vi "VisualMonitoring.vi"(8 "error in":errorcluster) -> ()   [LabVIEW 2014]
uses:
  Gantry/GantryGlobals.vi
  <vilib>/Rock Robotics/Network Tables/SD Write Numeric Array.vi
panel:
  out "Lift Setpoint":dbl
  out "Tote Sense 2":bool
  out "LiftSetpoint":dbl
  out "Gyro Angle":dbl
  out "Tote Sense":bool
  out "Front Left Wheel Encoder Position":dbl
  out "Front Left Wheel":dbl(graph)
  out "Right Arm Lift Velocity":dbl(graph)
  out "Left Arm Lift Velocity":dbl(graph)
  out "LiftError":dbl
  out "Closed Loop Error Gantry":dbl
  out "Closed Loop Error LiftL":dbl
  out "Closed Loop Error ArmR":dbl
  out "Closed Loop Error LiftR":dbl
  out "Closed Loop Error ArmL":dbl
  out "Left Arm Applied Throttle":dbl
  out "Right Arm Applied Throttle":dbl
  out "Encoder Position FL":dbl=414.0
  out "Applied Throttle FL":dbl
  out "Encoder Position FR":dbl=414.0
  out "Applied Throttle FR":dbl
  out "Encoder Position BL":dbl=414.0
  out "Applied Throttle BL":dbl
  out "Encoder Position BR":dbl=414.0
  out "Applied Throttle BR":dbl
  out "Closed Loop Error FL":dbl
  out "Closed Loop Error FR":dbl
  out "Closed Loop Error BL":dbl
  out "Closed Loop Error BR":dbl
  out "Right Lift":cluster{"FL Angle":dbl, "Encoder Position":dbl}(graph)={"FL Angle"=0.0, "Encoder Position"=1.0}
  out "Left Lift":cluster{"FL Angle":dbl, "Encoder Position":dbl}(graph)={"FL Angle"=2.0, "Encoder Position"=1.0}
  out "Gantry":cluster{"FL Angle":dbl, "Encoder Position":dbl}(graph)={"FL Angle"=2019.0, "Encoder Position"=2100.0}
  out "Left Arm":cluster{"FL Angle":dbl, "Encoder Position":dbl}(graph)
  out "Right Arm":cluster{"FL Angle":dbl, "Encoder Position":dbl}(graph)
  out "Gantry Position":dbl=2019.0
  out "Gantry Applied Throttle":dbl
  out "Lift Encoder R":dbl
  out "Lift Encoder L":dbl
  out "Right Lift Throttle":dbl
  out "Left Lift Throttle":dbl
  out "Left Arm Position":dbl
  out "Right Arm Position":dbl
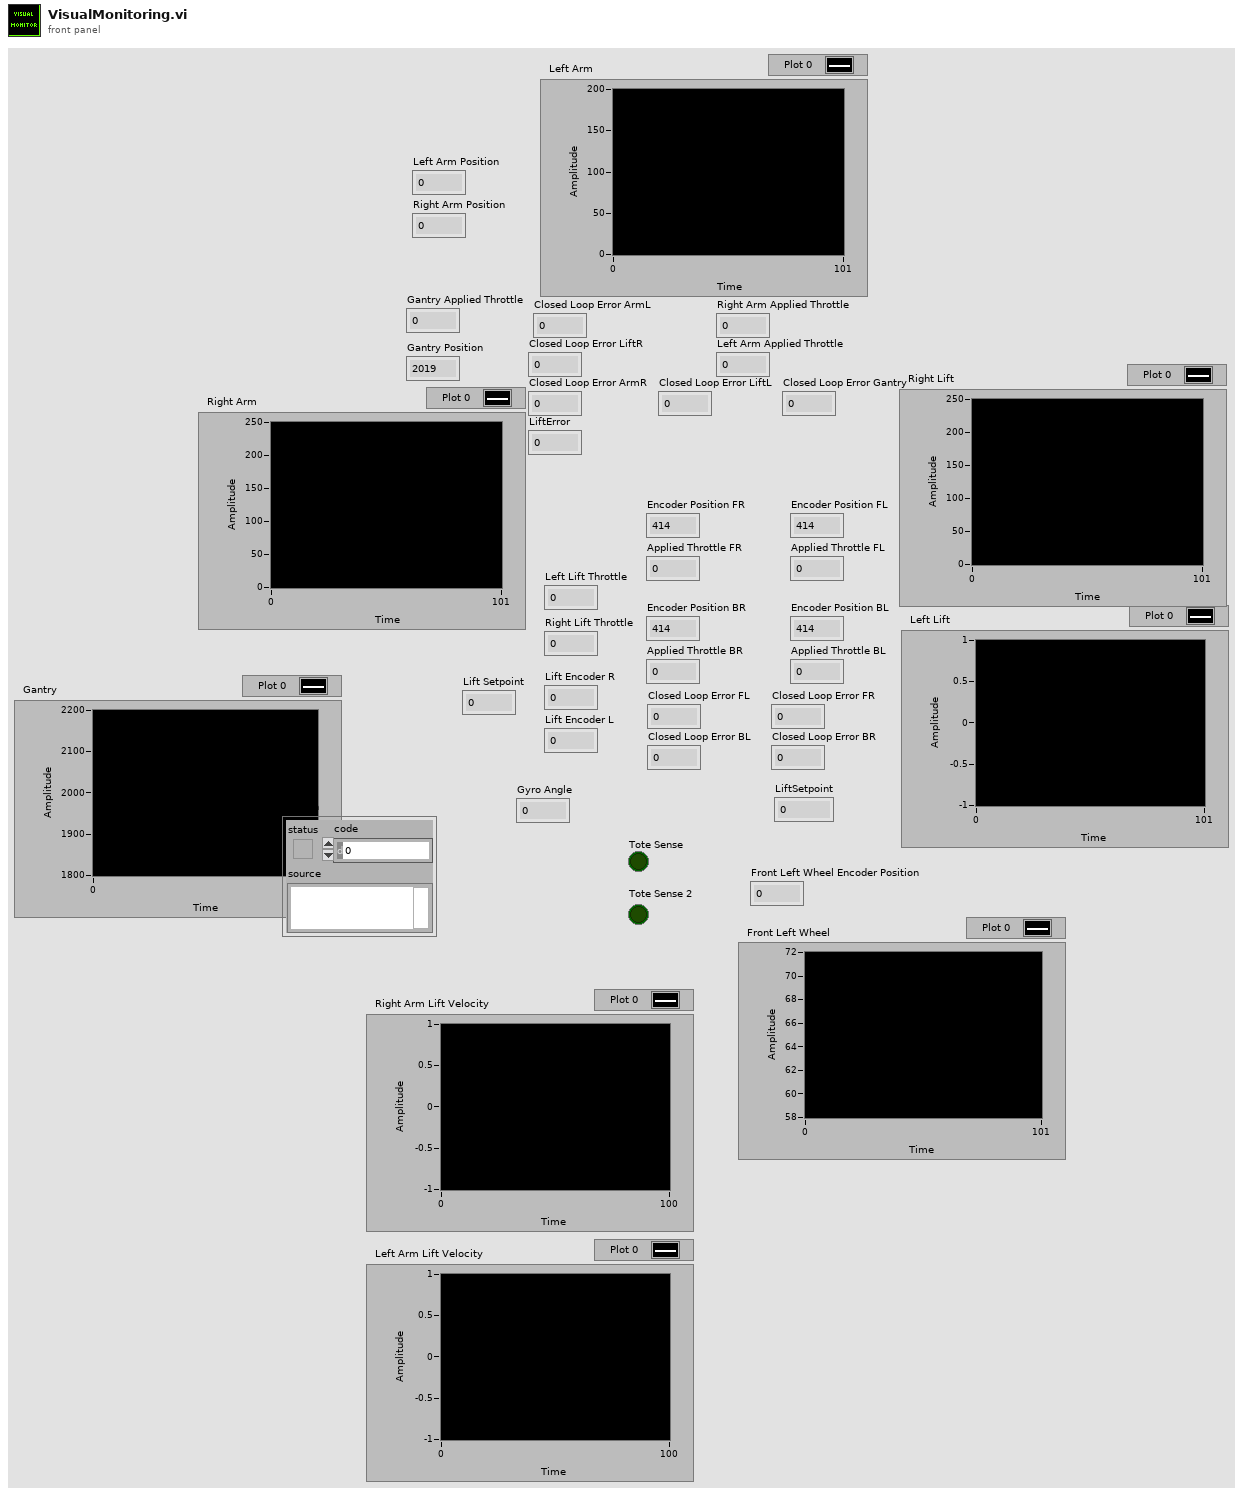
[diagram p1: front panel]
types:
  T1 = typedef "WPI_AccelerometerDevRef.ctl" = cluster{"DevStatus":errorcluster, "Controller":T2, "Scaling":T3, "Analog Channels":T4, "I2C Bus":T6, "SPI Bus":T7, "Accel Range":T8, "ADXL345 Axes":T9, "Handle":i32, "Device Address":u8, "Accel Type":enum16{"Analog", "ADXL345 I2C", "ADXL345 SPI", "Internal"}}
  T2 = typedef "FPGA_TypedefAnalogModule.ctl" = enum16{"Controller 1"}
  T3 = typedef "WPI_AccelerometerScaling.ctl" = cluster{"Gain (VoltsPerG)":dbl, "Center Voltage":dbl}
  T4 = typedef "WPI_AccelerometerAnalogChannels.ctl" = cluster{"X-Axis":T5, "Y-Axis":T5, "Z-Axis":T5}
  T5 = typedef "FPGA_AIChannel.ctl" = enum8{"AI 0", "AI 1", "AI 2", "AI 3", "AI MXP 0", "AI MXP 1", "AI MXP 2", "AI MXP 3", "Invalid"}
  T6 = typedef "i2c_bus.ctl" = enum16{"I2C On-Board", "I2C MXP", "Invalid"}
  T7 = typedef "spi_bus.ctl" = enum16{"SPI On-Board, CS0", "SPI On-Board, CS1", "SPI On-Board, CS2", "SPI On-Board, CS3", "SPI MXP", "Invalid"}
  T8 = typedef "ADXL345 Range.ctl" = u8
  T9 = typedef "WPI_AccelerometerADXL345 Axes.ctl" = cluster{"X-Axis":bool, "Y-Axis":bool, "Z-Axis":bool}
  T10 = cluster{"X-Axis":dbl, "Y-Axis":dbl, "Z-Axis":dbl}
  T11 = typedef "WPI_JoystickDevRef.ctl" = cluster{"Device":T12}
  T12 = typedef "WPI_JoystickDeviceEnum.ctl" = enum16{"USB 0", "USB 1", "USB 2", "USB 3", "USB 4", "USB 5"}
  T13 = typedef "WPI_SwitchDevRef.ctl" = cluster{"DevStatus":errorcluster, "DIO Channel":T14, "Controller":T15, "CntIndex":T16, "Normally Closed":bool}
  T14 = typedef "FPGA_DIOChannel.ctl" = enum8{"DIO 0", "DIO 1", "DIO 2", "DIO 3", "DIO 4", "DIO 5", "DIO 6", "DIO 7", "DIO 8", "DIO 9", "DIO MXP 0", "DIO MXP 1", "DIO MXP 2", "DIO MXP 3", "DIO MXP 4", "DIO MXP 5", "DIO MXP 6", "DIO MXP 7", "DIO MXP 8", "DIO MXP 9", "DIO MXP 10", "DIO MXP 11", "DIO MXP 12", "DIO MXP 13", "DIO MXP 14", "DIO MXP 15", "Invalid"}
  T15 = typedef "FPGA_TypedefDigitalModule.ctl" = enum16{"Controller 1"}
  T16 = typedef "FPGA_CounterCtrSystemIndex.ctl" = enum8{"Ctr 0", "Ctr 1", "Ctr 2", "Ctr 3", "Ctr 4", "Ctr 5", "Ctr 6", "Ctr 7", "Invalid"}
  T17 = typedef "WPI_GyroDevRef.ctl" = cluster{"DevStatus":errorcluster, "Analog Module":T2, "Analog Channel":T5, "Offset":dbl, "Gain (VoltsPerDegree/Second)":dbl}
  T18 = typedef "WPI_MotorControlDeviceRef.ctl" = cluster{"DeviceStatus":errorcluster, "Type":T19, "PWM":cluster{"Controller":T15, "PWM Channel":T20, "DeadBand":T21}, "CAN":cluster{"Device Number":u8, "Control Mode":T22, "Semaphore":T23, "Max Vout":dbl, "TalonSRX Control Mode":T24}, "Invert":bool, "TransformRef":T25, "InvTransformRef":T25}
  T19 = typedef "WPI_MotorControlType.ctl" = enum16{"PWM", "CAN", "CANTalonSRX"}
  T20 = typedef "FPGA_DIOPWMChannel.ctl" = enum8{"PWM 0", "PWM 1", "PWM 2", "PWM 3", "PWM 4", "PWM 5", "PWM 6", "PWM 7", "PWM 8", "PWM 9", "PWM MXP 0", "PWM MXP 1", "PWM MXP 2", "PWM MXP 3", "PWM MXP 4", "PWM MXP 5", "PWM MXP 6", "PWM MXP 7", "PWM MXP 8", "PWM MXP 9", "Invalid"}
  T21 = typedef "WPI_PWMDeadband.ctl" = cluster{"Name":string, "maxPositivePwm":i32, "minPositivePwm":i32, "centerPwm":i32, "maxNegativePwm":i32, "minNegativePwm":i32, "angularRange":u16}
  T22 = typedef "WPI_CANJaguar_ControlMode.ctl" = enum8{"Percent VBus", "Current", "Speed", "Position", "Voltage"}
  T23 = typedef "Semaphore RefNum" = refnum<k1>
  T24 = typedef "WPI_CANTalonSRX_APIControlMode.ctl" = enum8{"Percent VBus", "Speed", "Position", "Slave", "Unchanged / Invalid"}
  T25 = typedef "WPI_PWMTransform_ConPane.ctl" = refnum<vi>
  T26 = typedef "WPI_CANTalonSRX_GlobalStatus.ctl" = cluster{"Applied Throttle":dbl, "Module Enabled":bool, "CAN Error":errorcluster, "Closed Loop Error":dbl, "Forward Limit Switch Closed":bool, "Reverse Limit Switch Closed":bool, "Sensor Position":dbl, "Sensor Velocity":dbl, "Current":dbl, "Sticky Fault - Over Temp":bool, "Sticky Fault - Under Voltage":bool, "Sticky Fault - Forward Limit":bool, "Sticky Fault - Reverse Limit":bool, "Sticky Fault - Forward Soft Limit":bool, "Sticky Fault - Reverse Soft Limit":bool, "Brake is Enabled":bool, "Encoder Position":dbl, "Encoder Velocity":dbl, "Encoder Index Count":dbl, "Encoder A Pin State":bool, "Encoder B Pin State":bool, "Encoder Index Pin State":bool, "Analog In":dbl, "Analog In Velocity":dbl, "Temperature (C)":dbl, "Battery Voltage":dbl}
  T27 = cluster{"Encoder Position":dbl, "ArmSetpoint":dbl}
  T28 = cluster{"Encoder Position":dbl, "GantrySetpoint":dbl}
  T29 = cluster{"Encoder Position":dbl, "LiftSetpoint":dbl}
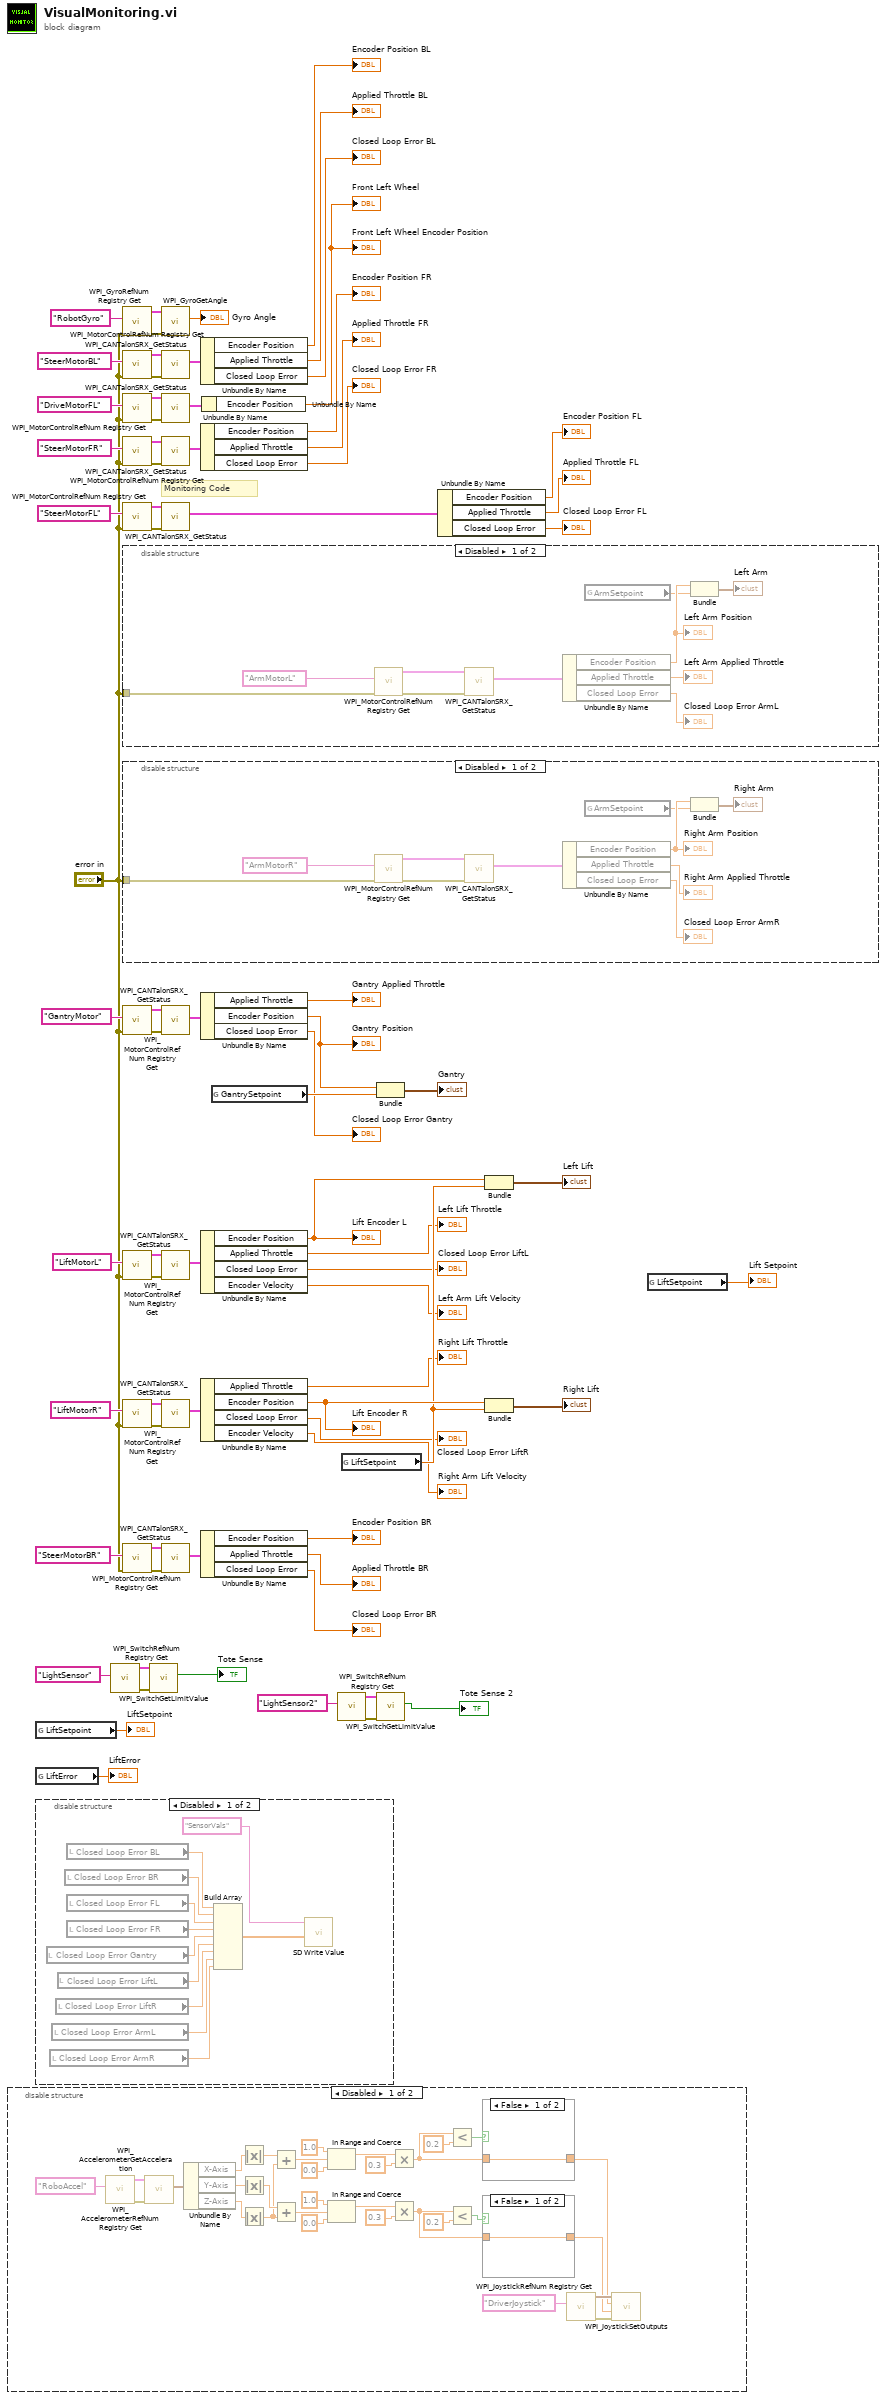
[diagram p0: block diagram]
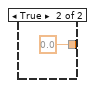
[diagram p2: hidden frame]
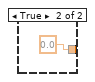
[diagram p3: hidden frame]
diagram:
  # "Monitoring Code"
  n1 = disable-structure shown="Disabled" {
    frame Disabled {
      n2 = call <vilib>:"WPI_AccelerometerRefNum Registry Get.vi"("refnum name"="RoboAccel") -> ("error out"=w107:errorcluster, "AccelerometerDevRef"=w106:T1)  [unwired: 9 in]
      n3 = call <vilib>:"WPI_AccelerometerGetAcceleration.vi"("error in"=w107, "AccelerometerDevRef"=w106) -> ("Accelerations"=w105:T10)  [unwired: 7 in, 2 out]
      n4 = Unbundle By Name(w105) -> ("X-Axis"=w101:dbl, "Y-Axis"=w100:dbl, "Z-Axis"=w99:dbl)
      n5 = Absolute Value(x=w101) -> (abs(x)=w92:dbl)
      n6 = Absolute Value(x=w100) -> (abs(x)=w91:dbl)
      n7 = Absolute Value(x=w99) -> (abs(x)=w90:dbl)
      n8 = Add(x=w92, y=w90) -> (x+y=w98:dbl)
      n9 = Add(x=w91, y=w90) -> (x+y=w93:dbl)
      n10 = In Range and Coerce(upper limit=1.0, x=w98, lower limit=0.0) -> (coerced(x)=w87:dbl)  [unwired: 1 out]
      n11 = In Range and Coerce(upper limit=1.0, x=w93, lower limit=0.0) -> (coerced(x)=w83:dbl)  [unwired: 1 out]
      n12 = Multiply(x=w87, y=0.3) -> (x*y=w81:dbl)
      n13 = Multiply(x=w83, y=0.3) -> (x*y=w79:dbl)
      n14 = Less?(x=w81, y=0.2) -> (x < y?=w88:bool)
      n15 = Less?(x=w79, y=0.2) -> (x < y?=w84:bool)
      n16 = case shown="False" w88 {
        tunnel: w81 -> [w111 _]
        tunnel: [w111 0.0 ("upper limit")] -> w86
        frame False {
        }
        frame True {
        }
      }
      n17 = case shown="False" w84 {
        tunnel: w79 -> [w109 _]
        tunnel: [w109 0.0 ("upper limit")] -> w82
        frame False {
        }
        frame True {
        }
      }
      n18 = call <vilib>:"WPI_JoystickRefNum Registry Get.vi"("refnum name"="DriverJoystick") -> ("error out"=w103:errorcluster, "JoystickDevRef"=w102:T11)  [unwired: 9 in]
      n19 = call <vilib>:"WPI_JoystickSetOutputs.vi"("error in (no error)"=w103, "Right Rumble"=w82, "Left Rumble"=w86, "JoystickDevRef"=w102) -> ()  [unwired: 6 in, 2 out]
    }
    frame Enabled {
    }
  }
  n20 = global read "GantryGlobals.vi" "LiftSetpoint"() -> (→"LiftSetpoint":dbl)
  n21 = global read "GantryGlobals.vi" "LiftError"() -> (→"LiftError":dbl)
  n22 = disable-structure shown="Disabled" {
    frame Disabled {
      n23 = local read "Closed Loop Error Gantry"() -> (w119:dbl)
      n24 = local read "Closed Loop Error ArmR"() -> (w115:dbl)
      n25 = local read "Closed Loop Error ArmL"() -> (w116:dbl)
      n26 = local read "Closed Loop Error LiftR"() -> (w117:dbl)
      n27 = local read "Closed Loop Error LiftL"() -> (w118:dbl)
      n28 = local read "Closed Loop Error BR"() -> (w122:dbl)
      n29 = local read "Closed Loop Error BL"() -> (w123:dbl)
      n30 = local read "Closed Loop Error FL"() -> (w121:dbl)
      n31 = local read "Closed Loop Error FR"() -> (w120:dbl)
      n32 = Build Array(w123, w122, w121, w120, w119, w118, w117, w116, w115) -> (w114:dbl[])
      n33 = call-poly <vilib>:"SD Write Value.vi"("Numeric Array"=w114, "Name"="SensorVals") -> ()  [unwired: 8 in, 2 out]
    }
    frame Enabled {
    }
  }
  n34 = call <vilib>:"WPI_SwitchRefNum Registry Get.vi"("refnum name"="LightSensor") -> ("error out"=w14:errorcluster, "SwitchDevRef"=w13:T13)  [unwired: 9 in]
  n35 = call <vilib>:"WPI_GyroRefNum Registry Get.vi"("error in (no error)"="error in", "refnum name"="RobotGyro") -> ("error out"=w10:errorcluster, "GyroDevRef"=w9:T17)  [unwired: 8 in]
  n36 = call <vilib>:"WPI_MotorControlRefNum Registry Get.vi"("error in (no error)"="error in", "refnum name"="SteerMotorBL") -> ("error out"=w69:errorcluster, "MotorControlDevRef"=w70:T18)  [unwired: 8 in]
  n37 = call <vilib>:"WPI_MotorControlRefNum Registry Get.vi"("error in (no error)"="error in", "refnum name"="DriveMotorFL") -> ("error out"=w18:errorcluster, "MotorControlDevRef"=w19:T18)  [unwired: 8 in]
  n38 = call <vilib>:"WPI_MotorControlRefNum Registry Get.vi"("error in (no error)"="error in", "refnum name"="SteerMotorFR") -> ("error out"=w72:errorcluster, "MotorControlDevRef"=w73:T18)  [unwired: 8 in]
  n39 = call <vilib>:"WPI_MotorControlRefNum Registry Get.vi"("error in (no error)"="error in", "refnum name"="SteerMotorFL") -> ("error out"=w75:errorcluster, "MotorControlDevRef"=w76:T18)  [unwired: 8 in]
  n40 = disable-structure shown="Disabled" {
    disable-tunnel: "error in" -> [w130 _]
    frame Disabled {
      n41 = call <vilib>:"WPI_MotorControlRefNum Registry Get.vi"("error in (no error)"=w130, "refnum name"="ArmMotorL") -> ("error out"=w131:errorcluster, "MotorControlDevRef"=w132:T18)  [unwired: 8 in]
      n42 = call <vilib>:"WPI_CANTalonSRX_GetStatus.vi"("error in (no error)"=w131, "CAN Talon SRX Ref"=w132) -> ("Talon SRX Status"=w129:T26)  [unwired: 7 in, 2 out]
      n43 = Unbundle By Name(w129) -> ("Encoder Position"=w128:dbl, "Applied Throttle"=→"Left Arm Applied Throttle":dbl, "Closed Loop Error"=→"Closed Loop Error ArmL":dbl)
      "Left Arm Position" <- w128
      n44 = global read "GantryGlobals.vi" "ArmSetpoint"() -> (w126:dbl)
      n45 = Bundle("Encoder Position"=w128, "ArmSetpoint"=w126) -> (→"Left Arm":T27)  [unwired: 1 in]
    }
    frame Enabled {
    }
  }
  n46 = disable-structure shown="Disabled" {
    disable-tunnel: "error in" -> [w134 _]
    frame Disabled {
      n47 = call <vilib>:"WPI_MotorControlRefNum Registry Get.vi"("error in (no error)"=w134, "refnum name"="ArmMotorR") -> ("error out"=w141:errorcluster, "MotorControlDevRef"=w142:T18)  [unwired: 8 in]
      n48 = call <vilib>:"WPI_CANTalonSRX_GetStatus.vi"("error in (no error)"=w141, "CAN Talon SRX Ref"=w142) -> ("Talon SRX Status"=w140:T26)  [unwired: 7 in, 2 out]
      n49 = Unbundle By Name(w140) -> ("Encoder Position"=w139:dbl, "Applied Throttle"=→"Right Arm Applied Throttle":dbl, "Closed Loop Error"=→"Closed Loop Error ArmR":dbl)
      "Right Arm Position" <- w139
      n50 = global read "GantryGlobals.vi" "ArmSetpoint"() -> (w135:dbl)
      n51 = Bundle("Encoder Position"=w139, "ArmSetpoint"=w135) -> (→"Right Arm":T27)  [unwired: 1 in]
    }
    frame Enabled {
    }
  }
  n52 = call <vilib>:"WPI_MotorControlRefNum Registry Get.vi"("error in (no error)"="error in", "refnum name"="GantryMotor") -> ("error out"=w57:errorcluster, "MotorControlDevRef"=w58:T18)  [unwired: 8 in]
  n53 = call <vilib>:"WPI_MotorControlRefNum Registry Get.vi"("error in (no error)"="error in", "refnum name"="LiftMotorL") -> ("error out"=w60:errorcluster, "MotorControlDevRef"=w61:T18)  [unwired: 8 in]
  n54 = call <vilib>:"WPI_MotorControlRefNum Registry Get.vi"("error in (no error)"="error in", "refnum name"="LiftMotorR") -> ("error out"=w63:errorcluster, "MotorControlDevRef"=w64:T18)  [unwired: 8 in]
  n55 = call <vilib>:"WPI_MotorControlRefNum Registry Get.vi"("error in (no error)"="error in", "refnum name"="SteerMotorBR") -> ("error out"=w66:errorcluster, "MotorControlDevRef"=w67:T18)  [unwired: 8 in]
  n56 = call <vilib>:"WPI_SwitchGetLimitValue.vi"("error in (no error)"=w14, "SwitchDevRef"=w13) -> ("Switch Pressed"=→"Tote Sense":bool)  [unwired: 7 in, 2 out]
  n57 = call <vilib>:"WPI_GyroGetAngle.vi"("error in (no error)"=w10, "GyroDevRef"=w9) -> ("Angle"=→"Gyro Angle":dbl)  [unwired: 6 in, 3 out]
  n58 = call <vilib>:"WPI_CANTalonSRX_GetStatus.vi"("error in (no error)"=w69, "CAN Talon SRX Ref"=w70) -> ("Talon SRX Status"=w51:T26)  [unwired: 7 in, 2 out]
  n59 = call <vilib>:"WPI_CANTalonSRX_GetStatus.vi"("error in (no error)"=w18, "CAN Talon SRX Ref"=w19) -> ("Talon SRX Status"=w17:T26)  [unwired: 7 in, 2 out]
  n60 = call <vilib>:"WPI_CANTalonSRX_GetStatus.vi"("error in (no error)"=w72, "CAN Talon SRX Ref"=w73) -> ("Talon SRX Status"=w54:T26)  [unwired: 7 in, 2 out]
  n61 = call <vilib>:"WPI_CANTalonSRX_GetStatus.vi"("error in (no error)"=w75, "CAN Talon SRX Ref"=w76) -> ("Talon SRX Status"=w56:T26)  [unwired: 7 in, 2 out]
  n62 = call <vilib>:"WPI_CANTalonSRX_GetStatus.vi"("error in (no error)"=w57, "CAN Talon SRX Ref"=w58) -> ("Talon SRX Status"=w33:T26)  [unwired: 7 in, 2 out]
  n63 = call <vilib>:"WPI_CANTalonSRX_GetStatus.vi"("error in (no error)"=w60, "CAN Talon SRX Ref"=w61) -> ("Talon SRX Status"=w39:T26)  [unwired: 7 in, 2 out]
  n64 = call <vilib>:"WPI_CANTalonSRX_GetStatus.vi"("error in (no error)"=w63, "CAN Talon SRX Ref"=w64) -> ("Talon SRX Status"=w40:T26)  [unwired: 7 in, 2 out]
  n65 = call <vilib>:"WPI_CANTalonSRX_GetStatus.vi"("error in (no error)"=w66, "CAN Talon SRX Ref"=w67) -> ("Talon SRX Status"=w48:T26)  [unwired: 7 in, 2 out]
  n66 = Unbundle By Name(w51) -> ("Encoder Position"=→"Encoder Position BL":dbl, "Applied Throttle"=→"Applied Throttle BL":dbl, "Closed Loop Error"=→"Closed Loop Error BL":dbl)
  n67 = Unbundle By Name(w54) -> ("Encoder Position"=→"Encoder Position FR":dbl, "Applied Throttle"=→"Applied Throttle FR":dbl, "Closed Loop Error"=→"Closed Loop Error FR":dbl)
  n68 = Unbundle By Name(w33) -> ("Applied Throttle"=→"Gantry Applied Throttle":dbl, "Encoder Position"=w30:dbl, "Closed Loop Error"=→"Closed Loop Error Gantry":dbl)
  "Gantry Position" <- w30
  n69 = Unbundle By Name(w39) -> ("Encoder Position"=w37:dbl, "Applied Throttle"=→"Left Lift Throttle":dbl, "Closed Loop Error"=→"Closed Loop Error LiftL":dbl, "Encoder Velocity"=→"Left Arm Lift Velocity":dbl)
  "Lift Encoder L" <- w37
  n70 = Unbundle By Name(w40) -> ("Applied Throttle"=→"Right Lift Throttle":dbl, "Encoder Position"=w38:dbl, "Closed Loop Error"=→"Closed Loop Error LiftR":dbl, "Encoder Velocity"=→"Right Arm Lift Velocity":dbl)
  "Lift Encoder R" <- w38
  n71 = Unbundle By Name(w48) -> ("Encoder Position"=→"Encoder Position BR":dbl, "Applied Throttle"=→"Applied Throttle BR":dbl, "Closed Loop Error"=→"Closed Loop Error BR":dbl)
  n72 = Unbundle By Name(w17) -> ("Encoder Position"=→"Front Left Wheel" →"Front Left Wheel Encoder Position":dbl)
  n73 = global read "GantryGlobals.vi" "GantrySetpoint"() -> (w32:dbl)
  n74 = call <vilib>:"WPI_SwitchRefNum Registry Get.vi"("refnum name"="LightSensor2") -> ("error out"=w4:errorcluster, "SwitchDevRef"=w3:T13)  [unwired: 9 in]
  n75 = global read "GantryGlobals.vi" "LiftSetpoint"() -> (w36:dbl)
  n76 = Bundle("Encoder Position"=w30, "GantrySetpoint"=w32) -> (→"Gantry":T28)  [unwired: 1 in]
  n77 = call <vilib>:"WPI_SwitchGetLimitValue.vi"("error in (no error)"=w4, "SwitchDevRef"=w3) -> ("Switch Pressed"=→"Tote Sense 2":bool)  [unwired: 7 in, 2 out]
  n78 = Unbundle By Name(w56) -> ("Encoder Position"=→"Encoder Position FL":dbl, "Applied Throttle"=→"Applied Throttle FL":dbl, "Closed Loop Error"=→"Closed Loop Error FL":dbl)
  n79 = Bundle("Encoder Position"=w37, "LiftSetpoint"=w36) -> (→"Left Lift":T29)  [unwired: 1 in]
  n80 = Bundle("Encoder Position"=w38, "LiftSetpoint"=w36) -> (→"Right Lift":T29)  [unwired: 1 in]
  n81 = global read "GantryGlobals.vi" "LiftSetpoint"() -> (→"Lift Setpoint":dbl)
